vi "A x Vector (Optimized).vi"(2 "Vector":dbl[](array[numeric]) format="%.2f", 3 "A":T1) -> (0 "error":i32, 1 "A x Vector":dbl[](array[numeric]) format="%.2f")   [LabVIEW 2014, in "NI_AALBase.lvlib"]
uses:
  NI_AALBase.lvlib
  RealMatrix.ctl
  lvanlys.dll
  NI_Matrix.lvlib
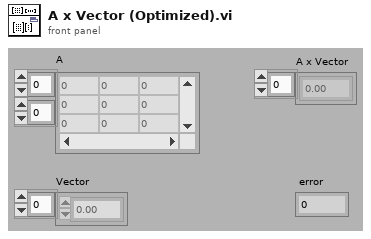
[diagram p1: front panel]
types:
  T1 = typedef "NI_Matrix.lvlib/RealMatrix.ctl" = dbl[][]
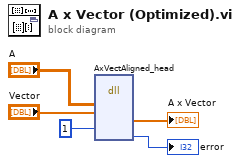
[diagram p0: block diagram]
diagram:
  n1 = dll-call lib="C:/Program Files (x86)/National Instruments/LabVIEW 2014/resource/lvanlys.*" fn="AxVectAligned_head"("aHandle"="A", "xHandle"="Vector", "isAligned"=1) -> ("yHandle"=→"A x Vector":dbl[], "dsperr"=→"error":i32)  [unwired: 9 in, 2 out]
